vi "App Config Path.vi"() -> (2 "App Config Path":path)   [LabVIEW 2015, in "App Config.lvlib"]
uses:
  App Config.lvlib
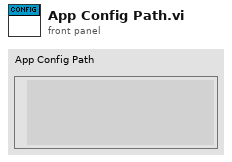
[diagram p1: front panel]
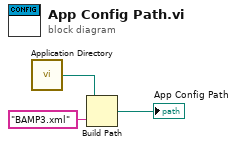
[diagram p0: block diagram]
diagram:
  n1 = call <vilib>:"Application Directory.vi"() -> ("Application Directory"=w3:path)
  n2 = Build Path(base path=w3, name or relative path="BAMP3.xml") -> (appended path=→"App Config Path":path)
